vi "SSS_V2.0.vi"() -> ()   [LabVIEW 2017]
uses:
  <vilib>/DAQmx/write.llb/DAQmx Write (Analog Wfm 1Chan NSamp).vi
  <vilib>/DAQmx/read.llb/DAQmx Read (Analog 1D Wfm NChan NSamp).vi
  <vilib>/measure/maspectr.llb/FFT Power Spectrum and PSD for 1 Chan.vi
  <vilib>/DAQmx/create/channels.llb/DAQmx Create Channel (AO-Voltage-Basic).vi
  <vilib>/DAQmx/configure/timing.llb/DAQmx Timing (Sample Clock).vi
  <vilib>/DAQmx/miscellaneous.llb/DAQmx Fill In Error Info.vi
  <vilib>/DAQmx/create/channels.llb/DAQmx Create Channel (AI-Voltage-Basic).vi
  <vilib>/Analysis/3filter.llb/FIR Filter (DBL).vi
  <vilib>/Analysis/NI_AALBase.lvlib
  <vilib>/measure/NI_MAPro.lvlib
panel:
  out "x-y":u32
  out "x-y 2":u32
  out "크기":i32
  out "Signal Processing Result 2":waveform(dbl)(graph)
  out "Pack(4byte)":string
  out "Signal Processing Result":waveform(dbl)(graph)
  out "RX.CH2":waveform(dbl)(graph)
  out "RX.CH1":waveform(dbl)(graph)
  in  "정지 버튼":bool
  in  "불리언":bool
  out "TX Spectrum":cluster{"f0":dbl, "df":dbl, "magnitude":dbl[]}(graph)
  out "TX Signal":waveform(dbl)(graph)
  in  "포트 번호":u16
  in  "주소":string
  in  "Pulse length(sec)":dbl=0.0004 format="%#_6p"
  in  "Stop Frequency(Hz)":dbl=470000.0 format="%#_6p"
  in  "Start Frequency(Hz)":dbl=430000.0 format="%#_6p"
  in  "송신 채널 설정":tag="Dev3/ao0"
  in  "송신 디바이스 이름":tag="Dev3"
  in  "Number of Sample":i32=150000
  in  "RX Time(sec)":dbl=2.0
  in  "수신 디바이스 이름":tag="Dev3"
  in  "수신 채널 설정":tag="Dev3/ai0:1"
  in  "sampling rate":dbl=1500000.0 caption="Sampling Frequency" format="%0.2f"
  in  "sample mode":i32(ring)=10123 caption="샘플 모드" items=["유한 샘플"=10178, "연속 샘플"=10123, "하드웨어 타이밍에 의한 단일 포인트"=12522]
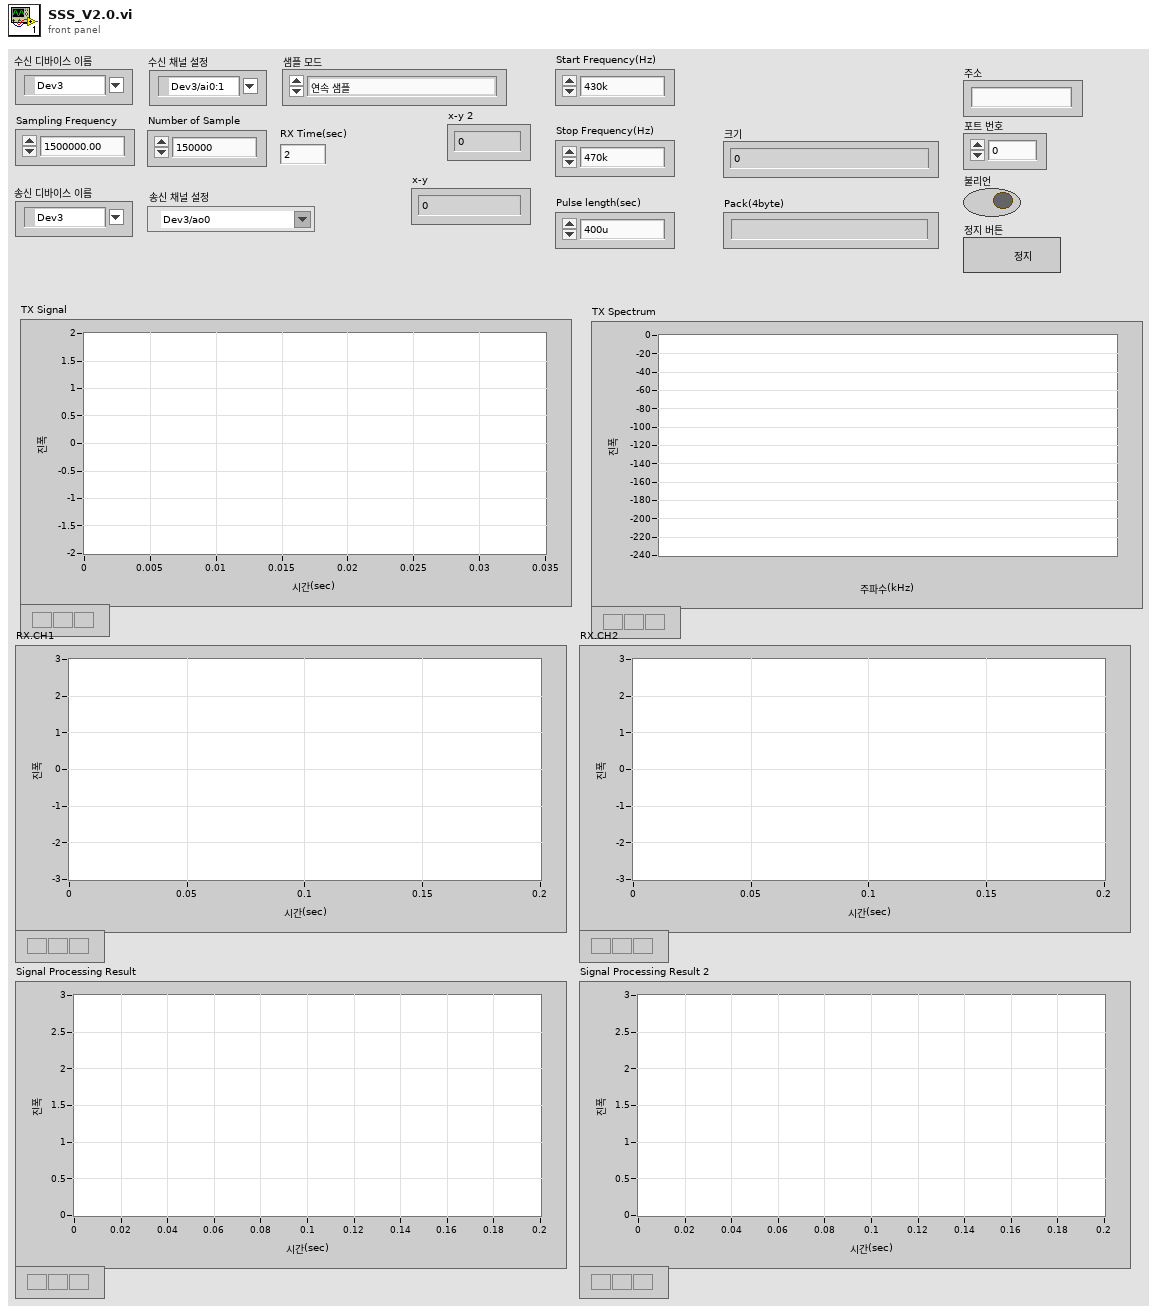
[diagram p1: front panel]
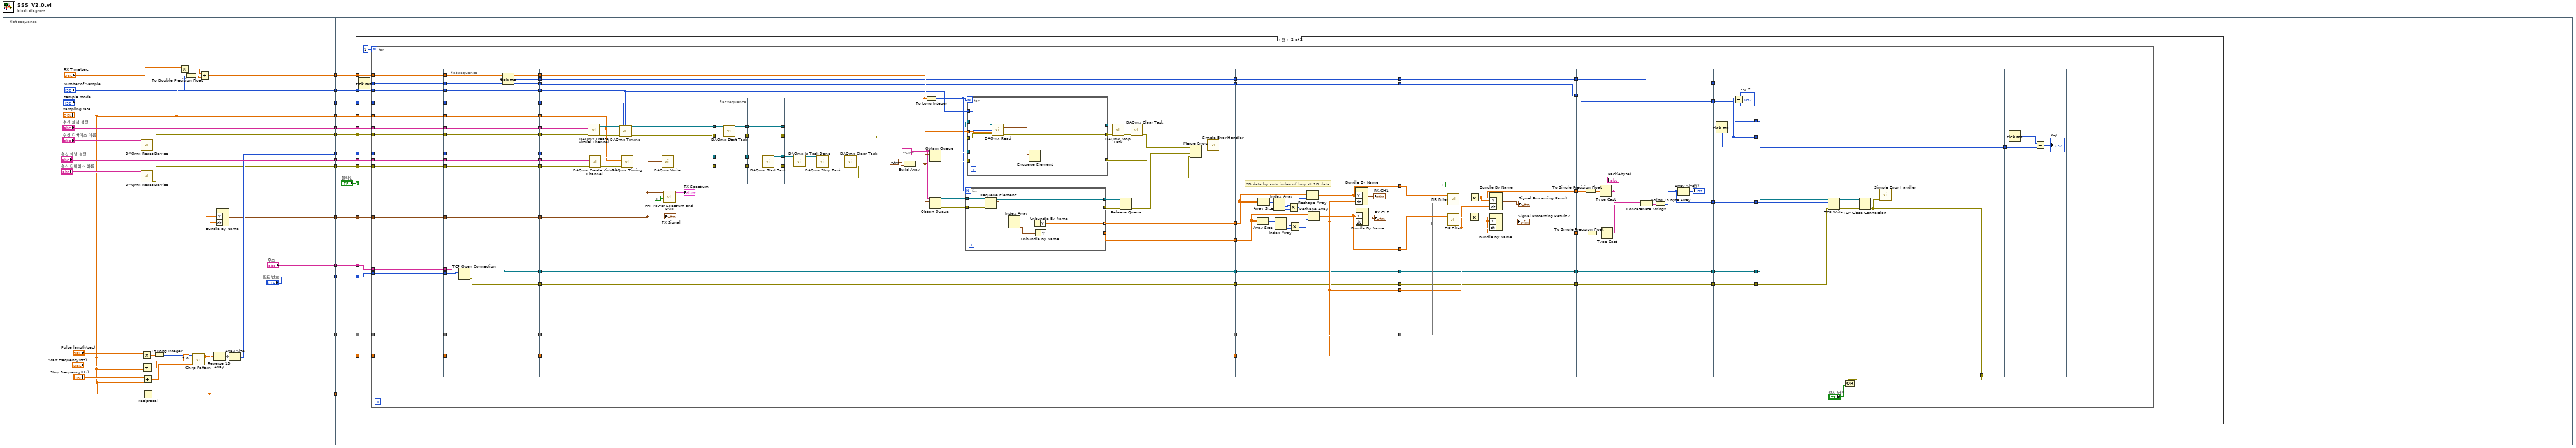
[diagram p0: block diagram]
diagram:
  n1 = flat-sequence {
    tunnel: ["수신 채널 설정"] -> w14
    tunnel: ["sampling rate"] -> w13
    tunnel: ["송신 채널 설정"] -> w12
    tunnel: ["sample mode"] -> w11
    tunnel: ["Number of Sample"] -> w10
    tunnel: [w29] -> w9
    tunnel: [w28] -> w8
    tunnel: [w27] -> w7
    tunnel: [w20] -> w6
    tunnel: [w21] -> w5
    tunnel: [w19] -> w4
    tunnel: [w18] -> w3
    tunnel: ["포트 번호"] -> w2
    tunnel: ["주소"] -> w1
    tunnel: w14 -> [w57]
    tunnel: w13 -> [w55]
    tunnel: w12 -> [w56]
    tunnel: w11 -> [w54]
    tunnel: w10 -> [w53]
    tunnel: w9 -> [w52]
    tunnel: w8 -> [w51]
    tunnel: w7 -> [w50]
    tunnel: w6 -> [w46]
    tunnel: w5 -> [w47]
    tunnel: w4 -> [w49]
    tunnel: w3 -> [w45]
    tunnel: w2 -> [w44]
    tunnel: w1 -> [w43]
    frame #0 {
      n2 = call <vilib>:"DAQmx Reset Device.vi"("device in"="수신 디바이스 이름") -> ("error out"=w28:errorcluster)  [unwired: 1 in, 13 out]
      n3 = call <vilib>:"DAQmx Reset Device.vi"("device in"="송신 디바이스 이름") -> ("error out"=w27:errorcluster)  [unwired: 1 in, 13 out]
      n4 = Multiply(x="Pulse length(sec)", y="sampling rate") -> (x*y=w41:dbl)
      n5 = Divide(x="Start Frequency(Hz)", y="sampling rate") -> (x/y=w38:dbl)
      n6 = Divide(x="Stop Frequency(Hz)", y="sampling rate") -> (x/y=w35:dbl)
      n7 = Reciprocal(x="sampling rate") -> (1/x=w20:dbl)
      n8 = To Long Integer(number=w41) -> (32bit integer=w40:i32)
      n9 = Multiply(x="RX Time(sec)", y="sampling rate") -> (x*y=w25:dbl)
      n10 = To Double Precision Float(number="Number of Sample") -> (double precision float=w26:dbl)
      n11 = call <vilib>:"Chirp Pattern.vi"("f2"=w35, "f1"=w38, "amplitude"=1.0, "samples"=w40) -> ("Chirp Pattern"=w15:dbl[])  [unwired: 1 out]
      n12 = Divide(x=w25, y=w26) -> (x/y=w21:dbl)
      n13 = Reverse 1D Array(array=w15) -> (reversed array=w18:dbl[])
      n14 = Bundle By Name("Y"=w15, "dt"=w20) -> (w19:waveform(dbl))  [unwired: 1 in]
      n15 = Array Size(array=w18) -> (size(s)=w29:i32)
    }
    frame #1 {
      n16 = case shown="참" "불리언" {
        tunnel: w57 -> [_ w73]
        tunnel: w56 -> [_ w72]
        tunnel: w55 -> [_ w71]
        tunnel: w54 -> [_ w70]
        tunnel: w53 -> [_ w69]
        tunnel: w52 -> [_ w68]
        tunnel: w51 -> [_ w67]
        tunnel: w50 -> [_ w66]
        tunnel: w49 -> [_ w65]
        tunnel: w47 -> [_ w64]
        tunnel: w46 -> [_ w63]
        tunnel: w45 -> [_ w62]
        tunnel: w44 -> [_ w61]
        tunnel: w43 -> [_ w60]
        frame False {
        }
        frame True {
          n17 = Tick Count (ms)() -> (millisecond timer value=w58:u32)
          n18 = for {
            N: 1 -> [_]
            tunnel: w73 -> [w139]
            tunnel: w72 -> [w138]
            tunnel: w71 -> [w137]
            tunnel: w70 -> [w136]
            tunnel: w69 -> [w130]
            tunnel: w68 -> [w135]
            tunnel: w67 -> [w134]
            tunnel: w66 -> [w133]
            tunnel: w65 -> [w132]
            tunnel: w64 -> [w131]
            tunnel: w63 -> [w127]
            tunnel: w62 -> [w123]
            tunnel: w61 -> [w104]
            tunnel: w60 -> [w103]
            tunnel: w58 -> [w80]
            n19 = flat-sequence {
              tunnel: w123 -> [w146]
              tunnel: w127 -> [w147]
              tunnel: w130 -> [w148]
              tunnel: w131 -> [w149]
              tunnel: w132 -> [w150]
              tunnel: w133 -> [w151]
              tunnel: w134 -> [w152]
              tunnel: w135 -> [w153]
              tunnel: w136 -> [w154]
              tunnel: w137 -> [w155]
              tunnel: w138 -> [w156]
              tunnel: w139 -> [w157]
              tunnel: [w157] -> w117
              tunnel: [w156] -> w116
              tunnel: [w155] -> w115
              tunnel: [w154] -> w114
              tunnel: [w153] -> w113
              tunnel: [w152] -> w112
              tunnel: [w151] -> w111
              tunnel: [w150] -> w110
              tunnel: [w149] -> w109
              tunnel: [w148] -> w108
              tunnel: [w147] -> w107
              tunnel: [w146] -> w106
              tunnel: w104 -> [w145]
              tunnel: w103 -> [w144]
              tunnel: [w143] -> w99
              tunnel: [w142] -> w95
              tunnel: [w141] -> w85
              tunnel: w80 -> [w141]
              tunnel: [w140] -> w75
              tunnel: [w171] -> w129
              tunnel: [w170] -> w128
              tunnel: [w169] -> w126
              tunnel: [w168] -> w121
              tunnel: w117 -> [w214]
              tunnel: w116 -> [w211]
              tunnel: w115 -> [w208]
              tunnel: w114 -> [w207]
              tunnel: w113 -> [w206]
              tunnel: w112 -> [w205]
              tunnel: w111 -> [w204]
              tunnel: w110 -> [w162]
              tunnel: w109 -> [w173]
              tunnel: w108 -> [w172]
              tunnel: w107 -> [w169]
              tunnel: w106 -> [w168]
              tunnel: [w166] -> w100
              tunnel: w99 -> [w166]
              tunnel: [w165] -> w96
              tunnel: w95 -> [w165]
              tunnel: [w164] -> w86
              tunnel: w85 -> [w164]
              tunnel: [w163] -> w76
              tunnel: w75 -> [w163]
              tunnel: w129 -> [w259]
              tunnel: w128 -> [w258]
              tunnel: w126 -> [w254]
              tunnel: [w257] -> w125
              tunnel: [w256] -> w124
              tunnel: [w255] -> w122
              tunnel: w121 -> [w255]
              tunnel: [w254] -> w120
              tunnel: [w253] -> w101
              tunnel: w100 -> [w253]
              tunnel: [w252] -> w97
              tunnel: w96 -> [w252]
              tunnel: [w251] -> w87
              tunnel: w86 -> [w251]
              tunnel: [w250] -> w77
              tunnel: w76 -> [w250]
              tunnel: w125 -> [w281]
              tunnel: w124 -> [w280]
              tunnel: w122 -> [w278]
              tunnel: w120 -> [w277]
              tunnel: [w276] -> w119
              tunnel: [w274] -> w118
              tunnel: [w273] -> w102
              tunnel: w101 -> [w273]
              tunnel: [w272] -> w98
              tunnel: w97 -> [w272]
              tunnel: [w271] -> w88
              tunnel: w87 -> [w271]
              tunnel: [w270] -> w78
              tunnel: w77 -> [w270]
              tunnel: w119 -> [w296]
              tunnel: w118 -> [w294]
              tunnel: [w289] -> w94
              tunnel: [w287] -> w92
              tunnel: [w288] -> w90
              tunnel: w102 -> [w288]
              tunnel: w98 -> [w287]
              tunnel: w88 -> [w286]
              tunnel: [w286] -> w84
              tunnel: [w285] -> w79
              tunnel: w78 -> [w285]
              tunnel: w94 -> [w304]
              tunnel: [w304] -> w93
              tunnel: w92 -> [w303]
              tunnel: [w303] -> w91
              tunnel: w90 -> [w302]
              tunnel: [w302] -> w89
              tunnel: w84 -> [w298]
              tunnel: [w300] -> w82
              tunnel: w79 -> [w299]
              tunnel: [w298] -> w74
              tunnel: [w309] -> w83
              tunnel: w89 -> [w306]
              tunnel: w91 -> [w307]
              tunnel: w93 -> [w308]
              tunnel: w82 -> [_]
              tunnel: [w305] -> w81
              tunnel: w74 -> [w305]
              tunnel: w81 -> [w312]
              frame #0 {
                n20 = TCP Open Connection(address=w144, remote port or service name=w145) -> (connection ID=w142:refnum<k5>, error out=w143:errorcluster)  [unwired: 3 in]
                n21 = Tick Count (ms)() -> (millisecond timer value=w140:u32)
              }
              frame #1 {
                w179 = "SIG" ("이름(이름없음)")
                w182 = waveform(dbl) {"t0"=timestamp(0 s since 1904-01-01), "dt"=1.0, "Y"=[]} ("Waveform")
                n22 = call-poly <vilib>:"DAQmx Create Virtual Channel.vi"("physical channels"=w214, "error in"=w205) -> ("task out"=w213:refnum<k21>, "error out"=w212:errorcluster)  [unwired: 7 in, 5 out]
                n23 = call-poly <vilib>:"DAQmx Create Virtual Channel.vi"("physical channels"=w211, "error in"=w204) -> ("task out"=w210:refnum<k21>, "error out"=w209:errorcluster)  [unwired: 7 in, 5 out]
                n24 = call-poly <vilib>:"DAQmx Timing.vi"("task/channels in"=w213, "sample mode"=w207, "samples per channel"=w172, "rate"=w208, "error in"=w212) -> ("task out"=w198:refnum<k21>, "error out"=w199:errorcluster)  [unwired: 2 in, 7 out]
                n25 = call-poly <vilib>:"DAQmx Timing.vi"("task/channels in"=w210, "samples per channel"=w206, "rate"=w208, "error in"=w209) -> ("task out"=w203:refnum<k21>, "error out"=w202:errorcluster)  [unwired: 3 in, 7 out]
                n26 = call-poly <vilib>:"DAQmx Write.vi"("task/channels in"=w203, "data"=w162, "error in"=w202) -> ("task out"=w197:refnum<k21>, "error out"=w196:errorcluster)  [unwired: 10 in, 1 out]
                n27 = call-poly <vilib>:"FFT Power Spectrum and PSD.vi"("dB On (F)"=TRUE, "time signal"=w162) -> ("Power Spectrum / PSD"=→"TX Spectrum":cluster{"f0":dbl, "df":dbl, "magnitude":dbl[]})  [unwired: 6 in, 3 out]
                n28 = flat-sequence {
                  tunnel: w199 -> [w243]
                  tunnel: [w242] -> w218
                  tunnel: [w241] -> w217
                  tunnel: w198 -> [w240]
                  tunnel: w196 -> [w239]
                  tunnel: [w239] -> w216
                  tunnel: w197 -> [w238]
                  tunnel: [w238] -> w215
                  tunnel: w218 -> [w249]
                  tunnel: [w249] -> w174
                  tunnel: [w248] -> w175
                  tunnel: w217 -> [w248]
                  tunnel: w216 -> [w247]
                  tunnel: w215 -> [w246]
                  tunnel: [w245] -> w161
                  tunnel: [w244] -> w160
                  frame #0 {
                    n29 = call <vilib>:"DAQmx Start Task.vi"("task/channels in"=w240, "error in"=w243) -> ("task out"=w241:refnum<k21>, "error out"=w242:errorcluster)  [unwired: 12 in]
                  }
                  frame #1 {
                    n30 = call <vilib>:"DAQmx Start Task.vi"("task/channels in"=w246, "error in"=w247) -> ("task out"=w245:refnum<k21>, "error out"=w244:errorcluster)  [unwired: 12 in]
                  }
                }
                n31 = call <vilib>:"DAQmx Is Task Done.vi"("task/channels in"=w161, "error in"=w160) -> ("task out"=w159:refnum<k21>, "error out"=w158:errorcluster)  [unwired: 11 in, 1 out]
                n32 = call <vilib>:"DAQmx Stop Task.vi"("task/channels in"=w159, "error in"=w158) -> ("task out"=w195:refnum<k21>, "error out"=w194:errorcluster)  [unwired: 12 in]
                n33 = call <vilib>:"DAQmx Clear Task.vi"("task in"=w195, "error in"=w194) -> ("error out"=w167:errorcluster)  [unwired: 13 in]
                n34 = Build Array(w182, w182) -> (w181:waveform(dbl)[])
                n35 = To Long Integer(number=w173) -> (32bit integer=w180:i32)
                n36 = Obtain Queue(name (unnamed)=w179, element data type=w181) -> (queue out=w185:refnum<queue>, error out=w184:errorcluster)  [unwired: 3 in, 1 out]
                n37 = Obtain Queue(name (unnamed)=w179, element data type=w181) -> (queue out=w191:refnum<queue>, error out=w190:errorcluster)  [unwired: 3 in, 1 out]
                n38 = for {
                  N: w180 -> [_]
                  tunnel: w185 -> [w227]
                  tunnel: w184 -> [w226]
                  tunnel: [w225] -> w178
                  tunnel: [w223] -> w176
                  tunnel: [w220] -> w171 mode=indexing
                  tunnel: [w221] -> w170 mode=indexing
                  n39 = Dequeue Element(queue=w227, error in (no error)=w226) -> (queue out=w223:refnum<queue>, element=w224:waveform(dbl)[], error out=w225:errorcluster)  [unwired: 1 in, 1 out]
                  n40 = Index Array(array=w224) -> (element #1=w222:waveform(dbl), element #2=w219:waveform(dbl))  [unwired: 2 in]
                  n41 = Unbundle By Name(w222) -> ("Y"=w220:dbl[])
                  n42 = Unbundle By Name(w219) -> ("Y"=w221:dbl[])
                }
                n43 = for {
                  N: w180 -> [_]
                  tunnel: w191 -> [w237]
                  tunnel: w190 -> [w236]
                  tunnel: [w235] -> w188
                  tunnel: [w234] -> w187
                  tunnel: [w233] -> w186
                  tunnel: w175 -> [w231]
                  tunnel: w174 -> [w230]
                  tunnel: w172 -> [w229]
                  tunnel: w173 -> [w228]
                  n44 = call-poly <vilib>:"DAQmx Read.vi"("task/channels in"=w231, "number of samples per channel"=w229, "timeout"=w228, "error in"=w230) -> ("task out"=w234:refnum<k21>, "data"=w232:waveform(dbl)[], "error out"=w233:errorcluster)  [unwired: 9 out]
                  n45 = Enqueue Element(queue=w237, element=w232, error in (no error)=w236) -> (error out=w235:errorcluster)  [unwired: 1 in, 2 out]
                }
                n46 = call <vilib>:"DAQmx Stop Task.vi"("task/channels in"=w187, "error in"=w186) -> ("task out"=w192:refnum<k21>, "error out"=w193:errorcluster)  [unwired: 12 out]
                n47 = Release Queue(queue=w176, error in (no error)=w178) -> (error out=w177:errorcluster)  [unwired: 3 out]
                n48 = call <vilib>:"DAQmx Clear Task.vi"("task in"=w192, "error in"=w193) -> ("error out"=w189:errorcluster)  [unwired: 13 out]
                n49 = Merge Errors(w189, w188, w177, w167) -> (w183:errorcluster)
                n50 = call <vilib>:"Simple Error Handler.vi"("error in (no error)"=w183) -> ()  [unwired: 4 in, 5 out]
                "TX Signal" <- w162
              }
              frame #2 {
                # "2D data by auto index of loop -> 1D data"
                n51 = Array Size(array=w258) -> (size(s)=w262:i32[])
                n52 = Array Size(array=w259) -> (size(s)=w266:i32[])
                n53 = Index Array(array=w266) -> (element #1=w268:i32, element #2=w267:i32)  [unwired: 2 in]
                n54 = Index Array(array=w262) -> (element #1=w264:i32, element #2=w263:i32)  [unwired: 2 in]
                n55 = Multiply(x=w268, y=w267) -> (x*y=w269:i32)
                n56 = Multiply(x=w264, y=w263) -> (x*y=w265:i32)
                n57 = Reshape Array(w259, w269) -> (w257:dbl[])
                n58 = Reshape Array(w258, w265) -> (w256:dbl[])
                n59 = Bundle By Name("Y"=w257, "dt"=w254) -> (→"RX.CH1":waveform(dbl))  [unwired: 1 in]
                n60 = Bundle By Name("Y"=w256, "dt"=w254) -> (→"RX.CH2":waveform(dbl))  [unwired: 1 in]
              }
              frame #3 {
                w283 = TRUE ("init/cont (init:F)")
                n61 = call-poly <vilib>:"FIR Filter.vi"("init/cont (init:F)"=w283, "FIR Coefficients"=w278, "X"=w280) -> ("Filtered X"=w279:dbl[])  [unwired: 1 in, 1 out]
                n62 = call-poly <vilib>:"FIR Filter.vi"("init/cont (init:F)"=w283, "FIR Coefficients"=w278, "X"=w281) -> ("Filtered X"=w282:dbl[])  [unwired: 1 in, 1 out]
                n63 = Absolute Value(x=w279) -> (abs(x)=w274:dbl[])
                n64 = Absolute Value(x=w282) -> (abs(x)=w276:dbl[])
                n65 = Bundle By Name("Y"=w274, "dt"=w277) -> (→"Signal Processing Result 2":waveform(dbl))  [unwired: 1 in]
                n66 = Bundle By Name("Y"=w276, "dt"=w277) -> (→"Signal Processing Result":waveform(dbl))  [unwired: 1 in]
              }
              frame #4 {
                n67 = To Single Precision Float(number=w296) -> (single precision float=w297:sgl[])
                n68 = To Single Precision Float(number=w294) -> (single precision float=w295:sgl[])
                n69 = Type Cast(x=w297) -> (*(type *) &x=w293:string)  [unwired: 1 in]
                "Pack(4byte)" <- w293
                n70 = Type Cast(x=w295) -> (*(type *) &x=w292:string)  [unwired: 1 in]
                n71 = Concatenate Strings(w293, w292) -> (w291:string)
                n72 = String To Byte Array(string=w291) -> (unsigned byte array=w289:u8[])
                n73 = Array Size(array=w289) -> (size(s)=→"크기":i32)
              }
              frame #5 {
                n74 = Tick Count (ms)() -> (millisecond timer value=w300:u32)
                n75 = Subtract(x=w300, y=w299) -> (x-y=→"x-y 2":u32)
              }
              frame #6 {
                n76 = TCP Write(connection ID=w307, data in=w308, error in (no error)=w306) -> (connection ID out=w310:refnum<k5>, error out=w311:errorcluster)  [unwired: 1 in, 1 out]
                n77 = TCP Close Connection(connection ID=w310, error in (no error)=w311) -> (error out=w309:errorcluster)  [unwired: 1 in, 1 out]
                n78 = call <vilib>:"Simple Error Handler.vi"("error in (no error)"=w309) -> ()  [unwired: 4 in, 5 out]
              }
              frame #7 {
                n79 = Tick Count (ms)() -> (millisecond timer value=w313:u32)
                n80 = Subtract(x=w313, y=w312) -> (x-y=→"x-y":u32)
              }
            }
            n81 = Compound Arithmetic op=OR(w83, "정지 버튼") -> ()  [unwired: 1 out]
          }
        }
      }
    }
  }
